vi "Get Data.vi"(9 "Path Name":path=path "10 Ft", 10 "Path Folder Address":path) -> (0 "Commands":cluster{"Time (s)":dbl, T1, bool}[](array[cluster]), 1 "Angles":dbl[](array[numeric]), 2 "Velocity":dbl[](array[numeric]), 3 "Booleans":T3)   [LabVIEW 2019]
uses:
  Bordeaux/bordeaux-pathinator/Bordeaux/Command Stuff/Single Cmd Info.ctl
  <vilib>/picture/picture.llb/imagedata.ctl
panel:
  in  "?":cluster{"Time (s)":dbl, "Distance (ft)":dbl}
  in  "?":cluster{"x":dbl, "y":dbl, "th":dbl}[](array[cluster])
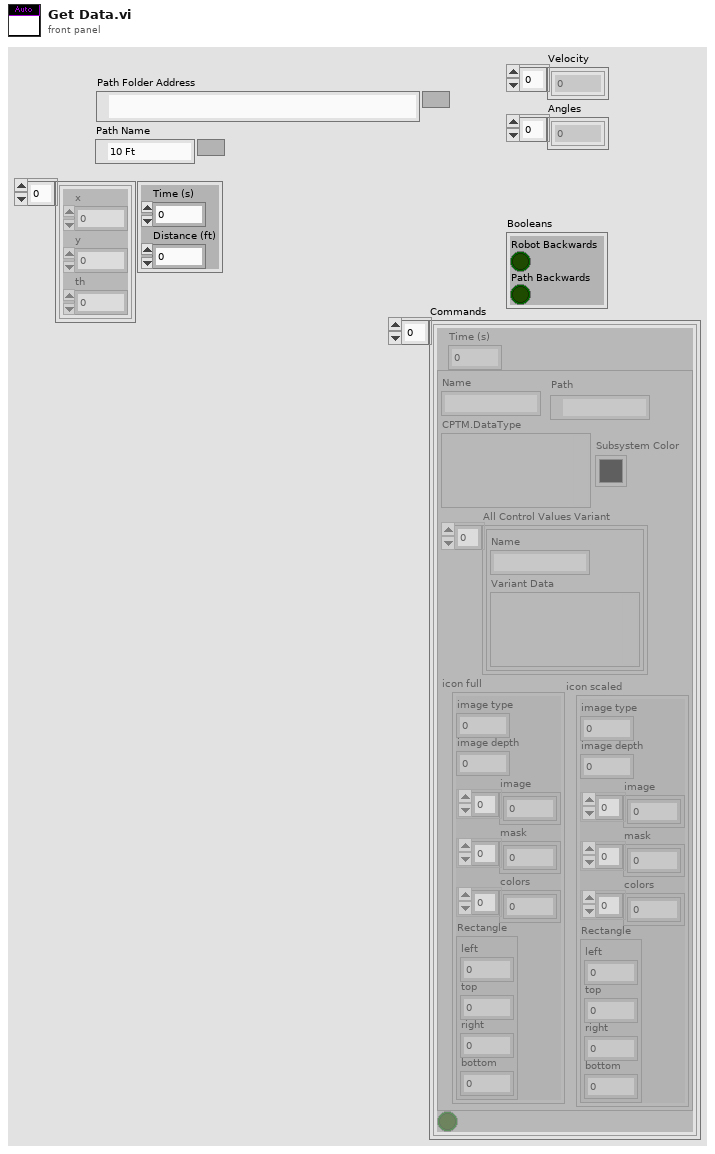
[diagram p1: front panel]
types:
  T1 = typedef "Single Cmd Info.ctl" = cluster{"Name":string, "CPTM.DataType":variant, "All Control Values Variant":cluster{"Name":string, "Variant Data":variant}[], "icon full":T2, "icon scaled":T2, "Path":path, "Subsystem Color":u32}
  T2 = typedef "imagedata.ctl" = cluster{"image type":i32, "image depth":i32, "image":u8[], "mask":u8[], "colors":u32[], "Rectangle":cluster{"left":i16, "top":i16, "right":i16, "bottom":i16}}
  T3 = cluster{"Robot Backwards":bool, "Path Backwards":bool}
  T4 = cluster{"Segment Name":string, "Type":enum16{"Accel Straight", "Const Straight", "Blend", "Circle"}, "Traj Pos Points":cluster{"x":dbl, "y":dbl, "th":dbl}[], "Traj Vel Points":cluster{"V":dbl, "th":dbl}[], "Accel Index":i32, "Decel Index":i32}[]
  T5 = cluster{"Sample Period (s)":dbl, "Limits":cluster{"Velocity (fps)":dbl, "Accel (fps^2)":dbl, "Turn Accel (fps^2)":dbl, "Jerk (fps^3)":dbl}, "Conditions":cluster{"vInitial (fps)":dbl, "vFinal (fps)":dbl}, cluster{dbl[], bool[]}}
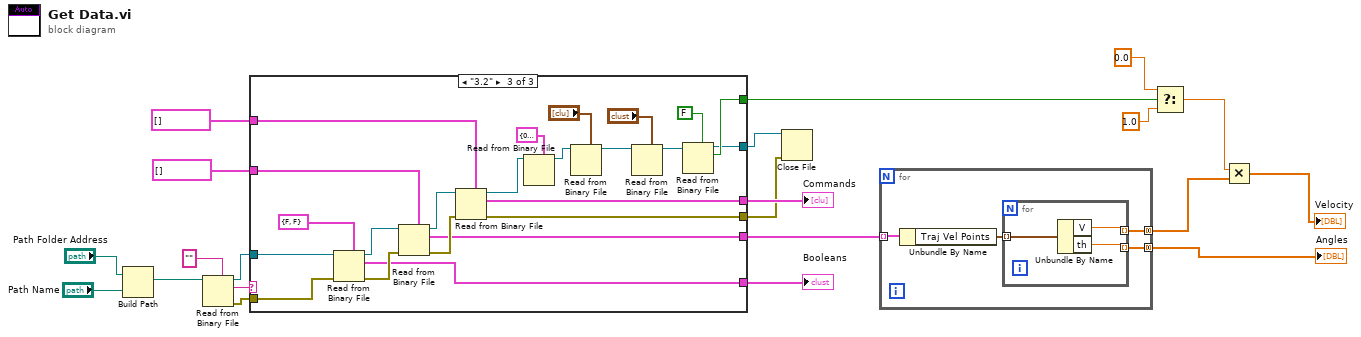
[diagram p0: block diagram]
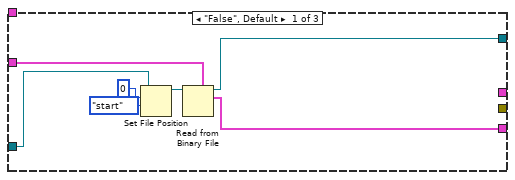
[diagram p2: hidden frame]
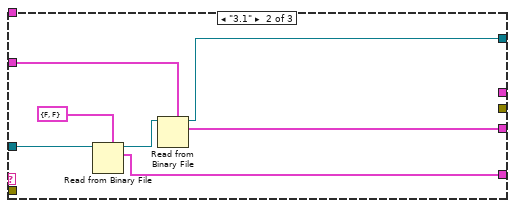
[diagram p3: hidden frame]
diagram:
  n1 = Build Path(base path="Path Folder Address", name or relative path="Path Name") -> (appended path=w15:path)
  n2 = Read from Binary File(5:"", 11:w15) -> (0:w8:errorcluster, 2:w20:string, 3:w19:refnum<file>)  [unwired: 4 in, 1 out]
  n3 = case shown="\"3.2\"" w20 {
    tunnel: w19 -> [w23 w34 w57]
    tunnel: T4 [] ("Trajectory Data") -> [w25 w35 w58]
    tunnel: [w24 w30 w47] -> w12
    tunnel: [w22 w31 w36] -> w18
    tunnel: [_ w29 w46] -> w13
    tunnel: cluster{"Time (s)":dbl, T1, bool}[] [] -> [_ _ w53]
    tunnel: [_ _ w48] -> w9
    tunnel: w8 -> [_ _ w52]
    tunnel: [_ _ w49] -> w7
    tunnel: [_ _ w37] -> w1
    frame "False", Default {
      n4 = Set File Position(offset (in bytes) (0)=i64 0, refnum=w23, from (0:start)=enum16{"start", "end", "current"}."start") -> (refnum out=w26:refnum<file>)  [unwired: 1 in, 1 out]
      n5 = Read from Binary File(5:w25, 11:w26) -> (2:w24:T4, 3:w22:refnum<file>)  [unwired: 4 in, 2 out]
    }
    frame "3.1" {
      n6 = Read from Binary File(5:cluster{bool, bool} {FALSE, FALSE} ("Cluster 2"), 11:w34) -> (2:w29:cluster{bool, bool}, 3:w32:refnum<file>)  [unwired: 4 in, 2 out]
      n7 = Read from Binary File(5:w35, 11:w32) -> (2:w30:T4, 3:w31:refnum<file>)  [unwired: 4 in, 2 out]
    }
    frame "3.2" {
      n8 = Read from Binary File(5:cluster{bool, bool} {FALSE, FALSE} ("Cluster 2"), 8:w52, 11:w57) -> (0:w51:errorcluster, 2:w46:cluster{bool, bool}, 3:w55:refnum<file>)  [unwired: 3 in, 1 out]
      n9 = Read from Binary File(5:w58, 8:w51, 11:w55) -> (0:w50:errorcluster, 2:w47:T4, 3:w54:refnum<file>)  [unwired: 3 in, 1 out]
      n10 = Read from Binary File(5:w53, 8:w50, 11:w54) -> (0:w49:errorcluster, 2:w48:cluster{"Time (s)":dbl, T1, bool}[], 3:w44:refnum<file>)  [unwired: 3 in, 1 out]
      n11 = Read from Binary File(5:T5 {"Sample Period (s)"=0.0, "Limits"={"Velocity (fps)"=0.0, "Accel (fps^2)"=0.0, "Turn Accel (fps^2)"=15.0, "Jerk (fps^3)"=0.0}, "Conditions"={"vInitial (fps)"=0.0, "vFinal (fps)"=0.0}, {[], []}} ("Cluster 2"), 11:w44) -> (3:w42:refnum<file>)  [unwired: 4 in, 3 out]
      n12 = Read from Binary File(5:"?", 11:w42) -> (3:w40:refnum<file>)  [unwired: 4 in, 3 out]
      n13 = Read from Binary File(5:"?", 11:w40) -> (3:w39:refnum<file>)  [unwired: 4 in, 3 out]
      n14 = Read from Binary File(5:FALSE, 11:w39) -> (2:w37:bool, 3:w36:refnum<file>)  [unwired: 4 in, 2 out]
    }
  }
  "Booleans" <- w13
  "Commands" <- w9
  n15 = Close File(refnum=w18, error in=w7) -> ()  [unwired: 2 out]
  n16 = for {
    tunnel: w12 -> [w62] mode=indexing
    tunnel: [w60] -> w6 mode=concatenating
    tunnel: [w59] -> w11 mode=concatenating
    n17 = Unbundle By Name(w62) -> ("Traj Vel Points"=w61:cluster{"V":dbl, "th":dbl}[])
    n18 = for {
      tunnel: w61 -> [w65] mode=indexing
      tunnel: [w64] -> w60 mode=indexing
      tunnel: [w63] -> w59 mode=indexing
      n19 = Unbundle By Name(w65) -> ("V"=w64:dbl, "th"=w63:dbl)
    }
  }
  "Angles" <- w11
  n20 = Select(t=0.0, s=w1, f=1.0) -> (s? t:f=w4:dbl)
  n21 = Multiply(x=w4, y=w6) -> (x*y=→"Velocity":dbl[])
